vi "RT_Rotation_Integration_v2 (SubVI).vi"(1 "W_b(i) [rad/s]":dbl[](array[numeric]), 2 "ang_acc [rad/s^2]":dbl[](array[numeric]), 4 "q(i) in":dbl[](array[numeric]), 7 "dt":dbl) -> (14 "W(i+1)":dbl[](array[numeric]), 16 "W_b(i+1) [rad/s]":dbl[](array[numeric]), 17 "q(i+1)":dbl[](array[numeric]), 19 "Euler angles (i+1) XYZ [rad]":dbl[](array[numeric]))   [LabVIEW 2017]
uses:
  <vilib>/Analysis/_algsub.llb/Vector Norm Type.ctl
  <vilib>/Analysis/coordinate.llb/Euler Rotation Order.ctl
  <vilib>/Analysis/baseanly.llb/Real A x B.vi
  <vilib>/Analysis/_algsub.llb/Real Vector Norm.vi
  <vilib>/Analysis/Matrix/Numeric/Conversions/Array To Matrix - RA.vi
  <vilib>/Analysis/Matrix/Numeric/Conversions/Array To Matrix - RA2.vi
  <vilib>/Analysis/Matrix/Numeric/Conversions/Matrix To Array - RM.vi
  <vilib>/Analysis/Matrix/NI_Matrix.lvlib
  <vilib>/Analysis/NI_AALBase.lvlib
  <vilib>/Analysis/NI_AALPro.lvlib
panel:
  out "Exp_Omega_k_T":dbl[][](array[numeric])
  out "S":dbl[][](array[numeric])
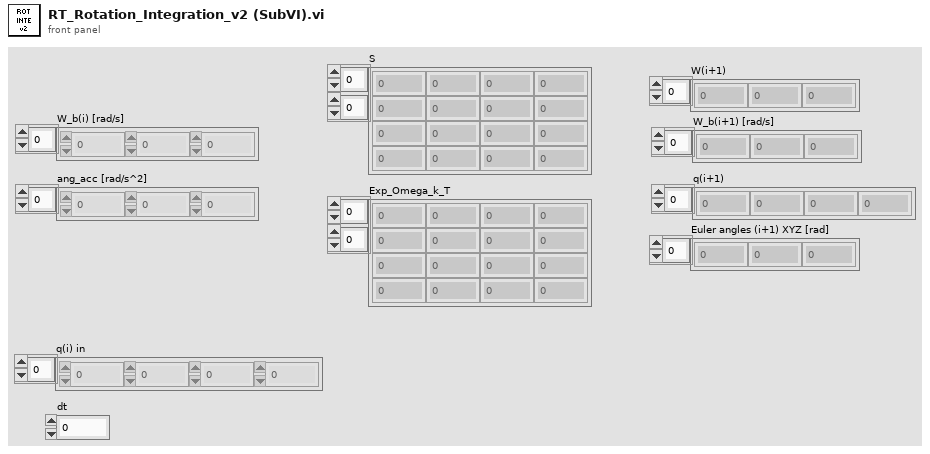
[diagram p1: front panel]
types:
  T1 = typedef "NI_AALPro.lvlib/Euler Rotation Order.ctl" = u16
  T2 = typedef "NI_AALPro.lvlib/Vector Norm Type.ctl" = u16
  T3 = typedef "NI_Matrix.lvlib/RealMatrix.ctl" = dbl[][]
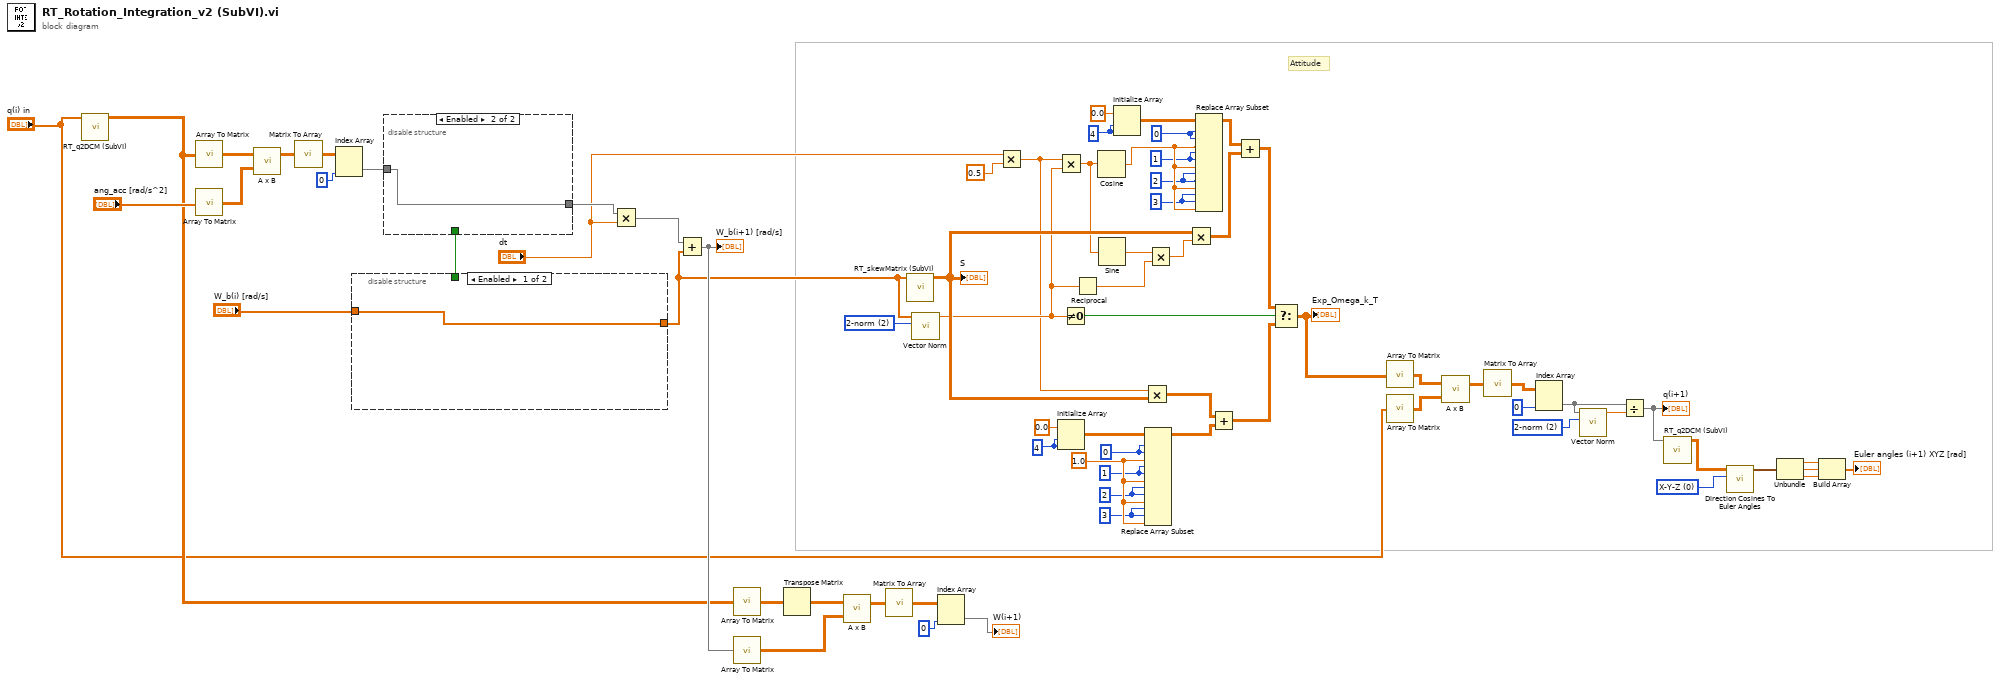
[diagram p0: block diagram]
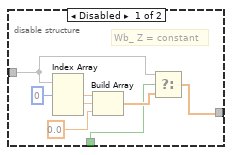
[diagram p2: hidden frame]
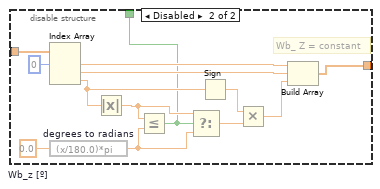
[diagram p3: hidden frame]
diagram:
  w26 = T1 0 items=["X-Y-Z", "X-Z-Y", "Y-X-Z", "Y-Z-X", "Z-X-Y", "Z-Y-X", "X-Y-X", "X-Z-X", "Y-X-Y", "Y-Z-Y", "Z-X-Z", "Z-Y-Z"] ("rotation order")
  w70 = T2 2 items=["1-norm"=1, "2-norm"=2, "Inf-norm"=3, "-Inf-norm"=4, "User Defined"=5] ("norm type")
  w59 = 1.0 ("new element/subarray")
  w54 = 3 ("disabled index (row)")
  w53 = 2 ("disabled index (row)")
  w52 = 1 ("disabled index (row)")
  w55 = 0 ("disabled index (row)")
  w58 = 4 ("dimension size")
  w47 = 3 ("disabled index (row)")
  w48 = 2 ("disabled index (row)")
  w49 = 1 ("disabled index (row)")
  w46 = 0 ("disabled index (row)")
  w36 = 4 ("dimension size")
  w34 = T2 2 items=["1-norm"=1, "2-norm"=2, "Inf-norm"=3, "-Inf-norm"=4, "User Defined"=5] ("norm type")
  # "Attitude"
  n1 = call "RT_q2DCM (SubVI).vi"("Quaternion"="q(i) in") -> ("DCM"=w6:dbl[][])  [unwired: 10 in]
  n2 = call-poly <vilib>:"Array To Matrix.vi"("Real 2D Array"=w6) -> ("Real Matrix"=w33:T3)
  n3 = call-poly <vilib>:"Array To Matrix.vi"("Real 1D Array"="ang_acc [rad/s^2]") -> ("Real Matrix (Column Vector)"=w32:T3)
  n4 = call-poly <vilib>:"A x B.vi"("B"=w32, "A"=w33) -> ("A x B"=w30:T3)  [unwired: 1 out]
  n5 = call-poly <vilib>:"Matrix To Array.vi"("Real Matrix"=w30) -> ("Real 2D Array"=w31:dbl[][])
  n6 = Index Array(array=w31, index (col)=0 ("index (row)")) -> (element=w9:dbl[])  [unwired: 1 in]
  n7 = disable-structure shown="Enabled" {
    disable-tunnel: [w73 w82] -> w1
    disable-tunnel: "W_b(i) [rad/s]" -> [w73 w85]
    disable-tunnel: [_ w74] -> w7
    frame Enabled {
    }
    frame Disabled {
      w81 = 0.0  # Wb_z [º]
      # "Wb_ Z = constant"
      n8 = Index Array(array=w85, index #1=0 ("index")) -> (element #1=w84:dbl, element #2=w83:dbl, element #3=w77:dbl)  [unwired: 2 in]
      n9 = expression code="(x/180.0)*pi" "degrees to radians"(w81) -> (w80:dbl)
      n10 = Absolute Value(x=w77) -> (abs(x)=w79:dbl)
      n11 = Less Or Equal?(x=w79, y=w80) -> (x <= y?=w74:bool)
      n12 = Select(t=w79, s=w74, f=w80) -> (s? t:f=w78:dbl)
      n13 = Sign(1:w77) -> (0:w76:dbl)
      n14 = Multiply(x=w76, y=w78) -> (x*y=w75:dbl)
      n15 = Build Array(w84, w83, w75) -> (w82:dbl[])
    }
  }
  n16 = disable-structure shown="Enabled" {
    disable-tunnel: w9 -> [w90 w95]
    disable-tunnel: [w88 w95] -> w8
    disable-tunnel: w7 -> [w87 _]
    frame Disabled {
      # "Wb_ Z = constant"
      n17 = Index Array(array=w90, index #1=0 ("index")) -> (element #1=w93:dbl, element #2=w92:dbl)  [unwired: 2 in, 1 out]
      n18 = Build Array(w93, w92, 0.0 ("element")) -> (w89:dbl[])
      n19 = Select(t=w90, s=w87, f=w89) -> (s? t:f=w88:dbl[])
    }
    frame Enabled {
    }
  }
  n20 = Multiply(x=w8, y="dt") -> (x*y=w27:dbl[])
  n21 = Add(x=w27, y=w1) -> (x+y=w12:dbl[])
  "W_b(i+1) [rad/s]" <- w12
  n22 = call-poly <vilib>:"Array To Matrix.vi"("Real 2D Array"=w6) -> ("Real Matrix"=w13:T3)
  n23 = call-poly <vilib>:"Array To Matrix.vi"("Real 1D Array"=w12) -> ("Real Matrix (Column Vector)"=w15:T3)
  n24 = Transpose Matrix(1:w13) -> (0:w14:T3)
  n25 = call-poly <vilib>:"A x B.vi"("B"=w15, "A"=w14) -> ("A x B"=w17:T3)  [unwired: 1 out]
  n26 = call-poly <vilib>:"Matrix To Array.vi"("Real Matrix"=w17) -> ("Real 2D Array"=w16:dbl[][])
  n27 = call "RT_skewMatrix (SubVI).vi"("vector"=w1) -> ("skew matrix"=w60:dbl[][])  [unwired: 10 in]
  "S" <- w60
  n28 = call-poly <vilib>:"Vector Norm.vi"("norm type"=w34, "Input Vector"=w1) -> ("norm"=w39:dbl)  [unwired: 8 in, 1 out]
  n29 = Index Array(array=w16, index (col)=0 ("index (row)")) -> (element=→"W(i+1)":dbl[])  [unwired: 1 in]
  n30 = Multiply(x="dt", y=0.5) -> (x*y=w2:dbl)
  n31 = Multiply(x=w2, y=w39) -> (x*y=w38:dbl)
  n32 = Initialize Array(0.0 ("element"), w58, w58) -> (w56:dbl[][])
  n33 = Not Equal To 0?(x=w39) -> (x != 0?=w35:bool)
  n34 = Reciprocal(x=w39) -> (1/x=w41:dbl)
  n35 = Cosine(x=w38) -> (cos(x)=w50:dbl)
  n36 = Sine(x=w38) -> (sin(x)=w40:dbl)
  n37 = Initialize Array(0.0 ("element"), w36, w36) -> (w44:dbl[][])
  n38 = Multiply(x=w2, y=w60) -> (x*y=w61:dbl[][])
  n39 = Replace Array Subset(array=w56, new element #1=w59, index (row) #1=w55, index (col) #1=w55, new element #2=w59, index (row) #2=w52, index (col) #2=w52, new element #3=w59, index (row) #3=w53, index (col) #3=w53, new element #4=w59, index (row) #4=w54, index (col) #4=w54) -> (w62:dbl[][])
  n40 = Multiply(x=w40, y=w41) -> (x*y=w42:dbl)
  n41 = Multiply(x=w60, y=w42) -> (x*y=w43:dbl[][])
  n42 = Replace Array Subset(array=w44, new element #1=w50, index (row) #1=w46, index (col) #1=w46, new element #2=w50, index (row) #2=w49, index (col) #2=w49, new element #3=w50, index (row) #3=w48, index (col) #3=w48, new element #4=w50, index (row) #4=w47, index (col) #4=w47) -> (w45:dbl[][])
  n43 = Add ("Add.vi")(x=w61, y=w62) -> (x+y=w63:dbl[][])
  n44 = Add ("Add.vi")(x=w45, y=w43) -> (x+y=w51:dbl[][])
  n45 = Select(t=w51, s=w35, f=w63) -> (s? t:f=w69:dbl[][])
  "Exp_Omega_k_T" <- w69
  n46 = call-poly <vilib>:"Array To Matrix.vi"("Real 2D Array"=w69) -> ("Real Matrix"=w68:T3)
  n47 = call-poly <vilib>:"Array To Matrix.vi"("Real 1D Array"="q(i) in") -> ("Real Matrix (Column Vector)"=w67:T3)
  n48 = call-poly <vilib>:"A x B.vi"("B"=w67, "A"=w68) -> ("A x B"=w65:T3)  [unwired: 1 out]
  n49 = call-poly <vilib>:"Matrix To Array.vi"("Real Matrix"=w65) -> ("Real 2D Array"=w66:dbl[][])
  n50 = Index Array(array=w66, index (col)=0 ("index (row)")) -> (element=w72:dbl[])  [unwired: 1 in]
  n51 = call-poly <vilib>:"Vector Norm.vi"("norm type"=w70, "Input Vector"=w72) -> ("norm"=w71:dbl)  [unwired: 8 in, 1 out]
  n52 = Divide(x=w72, y=w71) -> (x/y=w21:dbl[])
  "q(i+1)" <- w21
  n53 = call "RT_q2DCM (SubVI).vi"("Quaternion"=w21) -> ("DCM"=w20:dbl[][])  [unwired: 10 in]
  n54 = call <vilib>:"Direction Cosines To Euler Angles.vi"("rotation order"=w26, "Direction Cosines"=w20) -> ("Euler Angles"=w23:cluster{"phi":dbl, "theta":dbl, "psi":dbl})  [unwired: 8 in, 1 out]
  n55 = Unbundle(w23) -> ("phi"=w25:dbl, "theta"=w24:dbl, "psi"=w22:dbl)
  n56 = Build Array(w25, w24, w22) -> (→"Euler angles (i+1) XYZ [rad]":dbl[])
